vi "CRC32 MPEG 2.vi"(8 "error in (no error)":errorcluster, 11 "data":u8[](array[numeric])) -> (0 "error out":errorcluster, 3 "crc":u8[](array[numeric]))   [LabVIEW 2020]
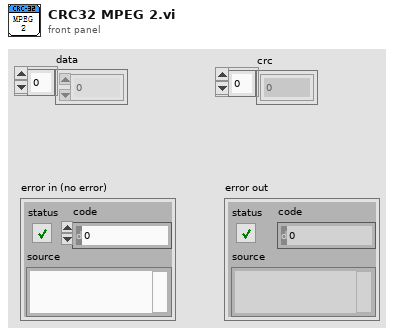
[diagram p1: front panel]
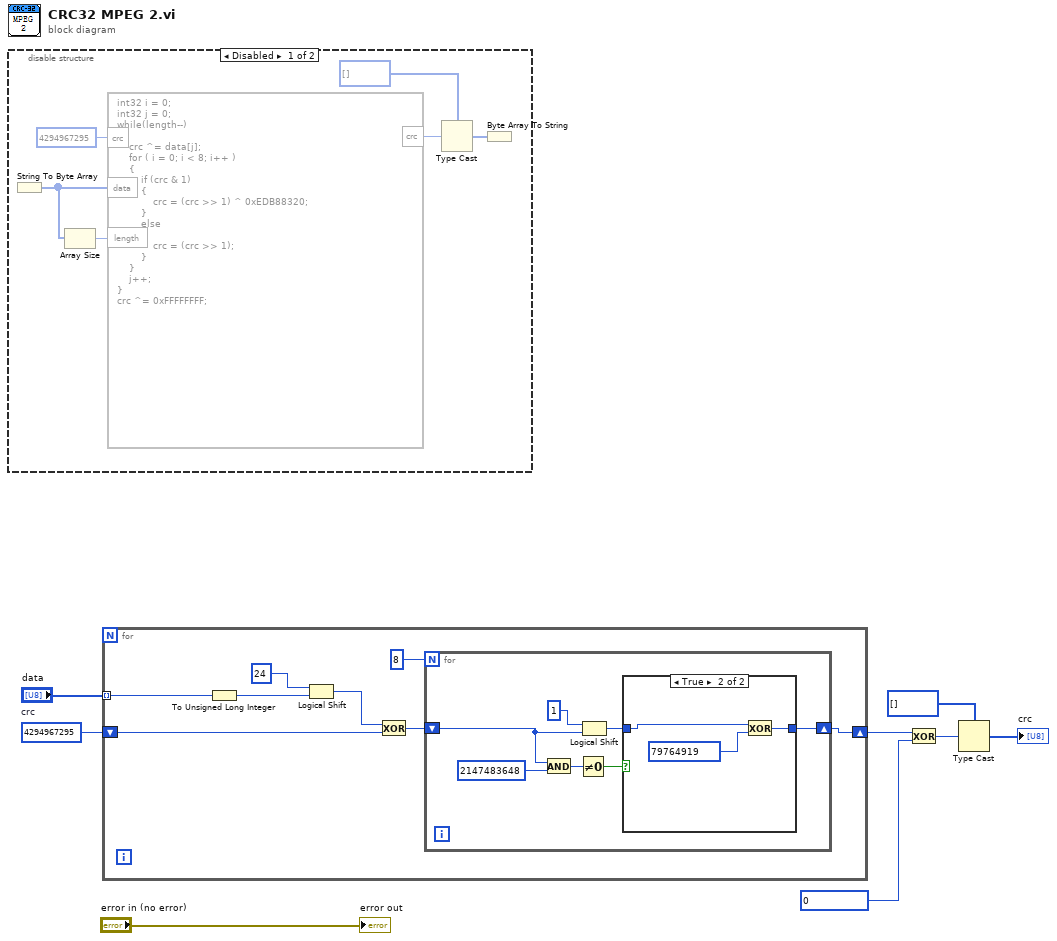
[diagram p0: block diagram]
diagram:
  w5 = u32 4294967295  # crc
  n1 = disable-structure shown="Disabled" {
    frame Disabled {
      n2 = String To Byte Array() -> (unsigned byte array=w14:u8[])  [unwired: 1 in]
      n3 = Array Size(array=w14) -> (size(s)=w13:i32)
      n4 = formula code="int32 i = 0;\nint32 j = 0;\nwhile(length--)\n{\n    crc ^= data[j]; \n    for ( i = 0; i < 8; i++ )\n    {\n        if (crc & 1)\n        {\n            crc = (crc >> 1) ^ 0xEDB88320;\n        }\n        else\n        {\n            crc = (crc >> 1);\n        }\n    }\n    j++;\n}\ncrc ^= 0xFFFFFFFF;"("data"=w14, "length"=w13, "crc"=u32 4294967295) -> ("crc"=w11:u32)
      n5 = Type Cast(type=u8[] [] ("unsigned byte array"), x=w11) -> (*(type *) &x=w9:u8[])
      n6 = Byte Array To String(unsigned byte array=w9) -> ()  [unwired: 1 out]
    }
    frame Enabled {
    }
  }
  n7 = for {
    shift-right: [w19] -> w6
    shift-left: w5 -> [w22]
    tunnel: "data" -> [w18] mode=indexing
    n8 = To Unsigned Long Integer(number=w18) -> (unsigned 32bit integer=w15:u32)
    n9 = Logical Shift(y=i16 24, x=w15) -> (x << y=w16:u32)
    n10 = Exclusive Or(1:w22, 2:w16) -> (0:w20:u32)
    n11 = for {
      N: 8 -> [_]
      shift-right: [w26] -> w19
      shift-left: w20 -> [w25]
      n12 = And(x=w25, y=u32 2147483648 ("x")) -> (x .and. y?=w28:u32)
      n13 = Not Equal To 0?(x=w28) -> (x != 0?=w27:bool)
      n14 = Logical Shift(y=i16 1, x=w25) -> (x << y=w24:u32)
      n15 = case shown="True" w27 {
        tunnel: [w30 w33] -> w26
        tunnel: w24 -> [w30 w32]
        frame False {
        }
        frame True {
          n16 = Exclusive Or(1:u32 79764919, 2:w32) -> (0:w33:u32)
        }
      }
    }
  }
  n17 = Exclusive Or(1:u32 0, 2:w6) -> (0:w4:u32)
  n18 = Type Cast(type=u8[] [] ("unsigned byte array"), x=w4) -> (*(type *) &x=→"crc":u8[])
  "error out" <- "error in (no error)"
